vi "Update States.vi"(8 "error in (no error)":errorcluster, 11 "Container in":refnum<class "Container.lvclass">) -> (0 "error out":errorcluster, 3 "Container out":refnum<class "Container.lvclass">)   [LabVIEW 2016, in "Container.lvclass"]
uses:
  Container.lvclass
  Container.lvclass/Container.ctl
  Sci/SciShutt.lvclass
  LFCSim/LFCSimShutt.lvclass
  ExtFlat/ExtFlatShutt.lvclass
  SimFlat/SimFlatShutt.lvclass
  Solar/CalShutt.lvclass
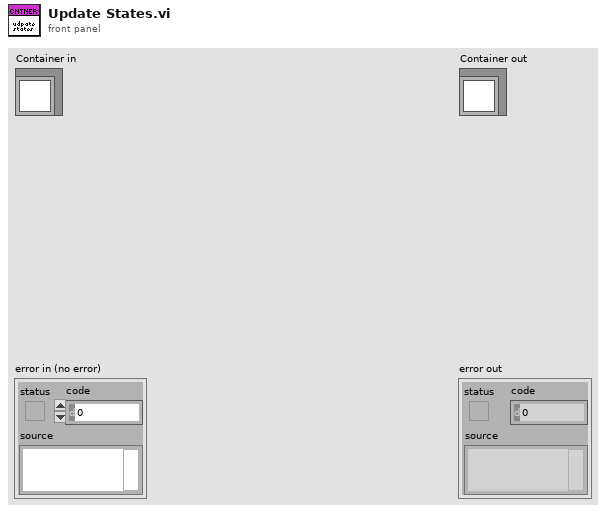
[diagram p1: front panel]
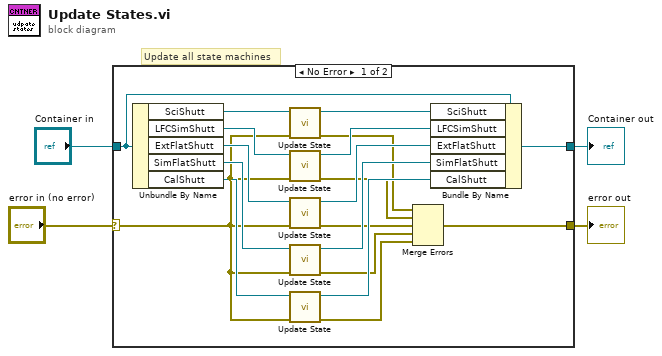
[diagram p0: block diagram]
diagram:
  # "Update all state machines"
  n1 = case shown="No Error" "error in (no error)" {
    selector: "error in (no error)" -> [w11 w25]
    tunnel: [w10 w25] -> w3
    tunnel: [w21 w24] -> w1
    tunnel: "Container in" -> [w22 w24]
    frame No Error {
      n2 = Unbundle By Name(w22) -> ("SciShutt"=w23:refnum<class "SciShutt.lvclass">, "LFCSimShutt"=w19:refnum<class "LFCSimShutt.lvclass">, "ExtFlatShutt"=w17:refnum<class "ExtFlatShutt.lvclass">, "SimFlatShutt"=w15:refnum<class "SimFlatShutt.lvclass">, "CalShutt"=w13:refnum<class "CalShutt.lvclass">)
      n3 = call-dynamic "Update State.vi"("error in (no error)"=w11, "BiStableShutter in"=w23) -> ("error out"=w9:errorcluster, "BiStableShutter out"=w20:refnum<class "SciShutt.lvclass">)  [unwired: 8 in]
      n4 = call-dynamic "Update State.vi"("error in (no error)"=w11, "UniStableShutter in"=w19) -> ("error out"=w8:errorcluster, "UniStableShutter out"=w18:refnum<class "LFCSimShutt.lvclass">)  [unwired: 8 in]
      n5 = call-dynamic "Update State.vi"("error in (no error)"=w11, "UniStableShutter in"=w17) -> ("error out"=w7:errorcluster, "UniStableShutter out"=w16:refnum<class "ExtFlatShutt.lvclass">)  [unwired: 8 in]
      n6 = call-dynamic "Update State.vi"("error in (no error)"=w11, "UniStableShutter in"=w15) -> ("error out"=w6:errorcluster, "UniStableShutter out"=w12:refnum<class "SimFlatShutt.lvclass">)  [unwired: 8 in]
      n7 = call-dynamic "Update State.vi"("error in (no error)"=w11, "UniStableShutter in"=w13) -> ("error out"=w5:errorcluster, "UniStableShutter out"=w14:refnum<class "CalShutt.lvclass">)  [unwired: 8 in]
      n8 = Merge Errors(w9, w8, w7, w6, w5) -> (w10:errorcluster)
      n9 = Bundle By Name(cluster=w22, "SciShutt"=w20, "LFCSimShutt"=w18, "ExtFlatShutt"=w16, "SimFlatShutt"=w12, "CalShutt"=w14) -> (w21:refnum<class "Container.lvclass">)
    }
    frame Error {
    }
  }
  "error out" <- w3
  "Container out" <- w1
